vi "Write All Elements GUI.vi"(8 "error in (no error)":errorcluster, 10 "Acquisition params.":T1={"Acquisition mode"=enum."Continuous", "Batch size"=50, "Image buffer size"=10, "Trigger mode"=enum."Framegrabber timed (sync.)", "Duration HH"=1.0, "Acquisition start"=enum."Immediate", "Duration SS"=0.0, "Duration MM"=0.0, "Start time"=timestamp(0 s since 1904-01-01), "Max. frame rate"=5.0, "Exposure time cam. 1"=1.0, "Exposure time cam. 2"=1.0, "Exposure mode"=enum."Linear", "Value 1"=17.0, "Value 2"=14.0, "Time 1"=1000.0, "Time 2"=1000.0} {"Exposure time cam. 2" min=0.01 step=0.01 format="%#.2g"; "Exposure time cam. 1" min=0.01 step=0.01 format="%#.2g"; "Max. frame rate" min=0.0001 max=1000000.0 format="%#.4g"; "Start time" format="%<%X\n%x>T"; "Duration MM" min=0 max=59 step=1 format="%02.0f"; "Duration SS" min=0 max=59 step=1 format="%02.0f"; "Duration HH" min=0 step=1 format="%02.0f"; "Image buffer size" min=1 max=10000 step=1 format="%#.0f"; "Batch size" min=1 max=50000 step=1}, 11 "Acquis params in":refnum<class "CV-Acquisition.lvclass">) -> (0 "error out":errorcluster, 3 "Acquis params out":refnum<class "CV-Acquisition.lvclass">)   [LabVIEW 2013, in "CameraVision.lvlib" / "CV-Acquisition.lvclass"]
uses:
  CV-Acquisition.lvclass
  Acquisition-parameters-gui.ctl
  Trigger-modes.ctl
  Exposure-modes.ctl
  CV-Acquisition.lvclass/CV-Acquisition.ctl
panel:
  # ":"
  # ":"
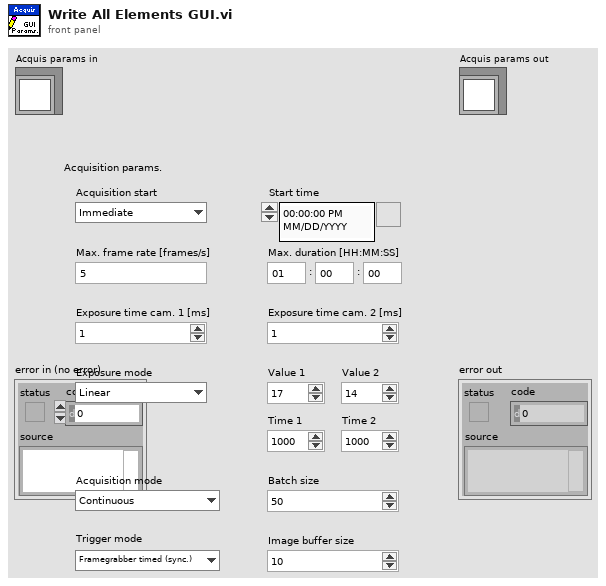
[diagram p1: front panel]
types:
  T1 = typedef "CameraVision.lvlib/CV-Acquisition.lvclass/Acquisition-parameters-gui.ctl" = cluster{"Acquisition mode":enum16{"Continuous", "Continuous batch", "Single batch", "Single batch -delayed"}, "Batch size":i32, "Image buffer size":i32, "Trigger mode":T2, "Duration HH":sgl, "Acquisition start":enum16{"Immediate", "Post-phoned"}, "Duration SS":sgl, "Duration MM":sgl, "Start time":timestamp, "Max. frame rate":dbl, "Exposure time cam. 1":dbl, "Exposure time cam. 2":dbl, "Exposure mode":T3, "Value 1":dbl, "Value 2":dbl, "Time 1":dbl, "Time 2":dbl}
  T2 = typedef "CameraVision.lvlib/CV-Acquisition.lvclass/Trigger-modes.ctl" = enum16{"Camera timed (not sync.)", "Framegrabber timed (sync.)", "Software timed (sync.)", "External timing (sync.)", "Manual (sync.)", "Gated - camera (not sync.)", "Gated - grabber (sync.)", "Gated - software (sync.)", "Gated - external (sync.)"}
  T3 = typedef "CameraVision.lvlib/CV-Acquisition.lvclass/Exposure-modes.ctl" = enum16{"Linear", "LinLog"}
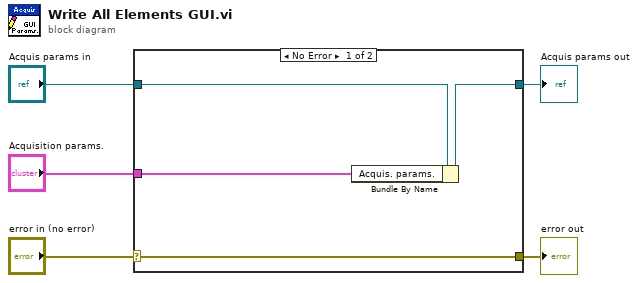
[diagram p0: block diagram]
diagram:
  n1 = case shown="No Error" "error in (no error)" {
    selector: "error in (no error)" -> [w9 w10]
    tunnel: [w9 w10] -> w4
    tunnel: [w7 w11] -> w2
    tunnel: "Acquis params in" -> [w8 w11]
    tunnel: "Acquisition params." -> [w6 _]
    frame No Error {
      n2 = Bundle By Name(cluster=w8, "Acquis. params."=w6) -> (w7:refnum<class "CV-Acquisition.lvclass">)
    }
    frame Error {
    }
  }
  "error out" <- w4
  "Acquis params out" <- w2
